vi "Create Rotated Ellipse.vi"(9 "aspect ratio":cluster{"x":dbl, "y":dbl}={"x"=1.0, "y"=0.8}, 11 "diameter points":T1) -> (3 "XY Graph":cluster{"X":dbl, "Y":dbl}[](graph))   [LabVIEW 2019]
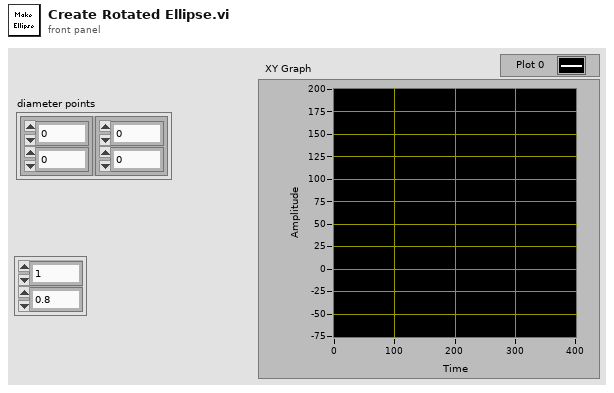
[diagram p1: front panel]
types:
  T1 = cluster{"first point":cluster{"x":dbl, "y":dbl}, "projected point":cluster{"x":dbl, "y":dbl}}
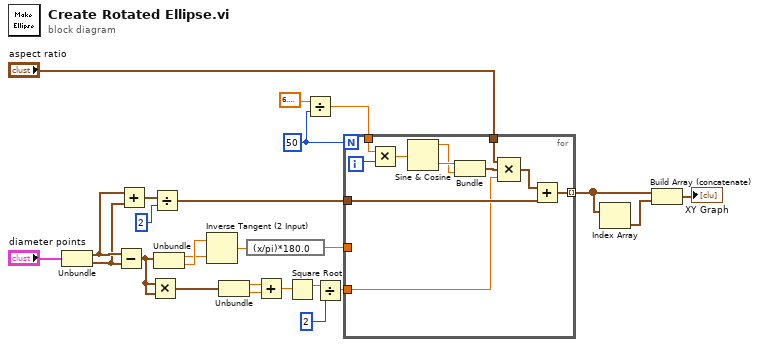
[diagram p0: block diagram]
diagram:
  w13 = 50
  n1 = Unbundle("diameter points") -> ("first point"=w22:cluster{"x":dbl, "y":dbl}, "projected point"=w21:cluster{"x":dbl, "y":dbl})
  n2 = Subtract(x=w22, y=w21) -> (x-y=w18:cluster{"x":dbl, "y":dbl})
  n3 = Add(x=w22, y=w21) -> (x+y=w20:cluster{"x":dbl, "y":dbl})
  n4 = Multiply(x=w18, y=w18) -> (x*y=w17:cluster{"x":dbl, "y":dbl})
  n5 = Divide(x=w20, y=2) -> (x/y=w15:cluster{"x":dbl, "y":dbl})
  n6 = Unbundle(w18) -> ("x"=w23:dbl, "y"=w24:dbl)
  n7 = Inverse Tangent (2 Input)(1:w23, 2:w24) -> (0:w3:dbl)
  n8 = Unbundle(w17) -> ("x"=w8:dbl, "y"=w7:dbl)
  n9 = expression code="(x/pi)*180.0" ("radians to degrees")(w3) -> (w2:dbl)
  n10 = Add(x=w8, y=w7) -> (x+y=w16:dbl)
  n11 = Square Root(x=w16) -> (sqrt(x)=w5:dbl)
  n12 = Divide(x=6.283185307179586, y=w13) -> (x/y=w12:dbl)
  n13 = Divide(x=w5, y=2) -> (x/y=w6:dbl)
  n14 = for {
    N: w13 -> [_]
    tunnel: w15 -> [w31]
    tunnel: w12 -> [w35]
    tunnel: [w30] -> w11 mode=indexing
    tunnel: w6 -> [w28]
    tunnel: w2 -> [_]
    tunnel: "aspect ratio" -> [w26]
    i -> [w36]
    n15 = Multiply(x=w35, y=w36) -> (x*y=w34:dbl)
    n16 = Sine & Cosine(0:w34) -> (1:w32:dbl, 2:w33:dbl)
    n17 = Bundle(w33, w32) -> (w29:cluster{dbl, dbl})  [unwired: 1 in]
    n18 = Compound Arithmetic op=MULTIPLY(w26, w29, w28) -> (w27:cluster{dbl, dbl})
    n19 = Add(x=w27, y=w31) -> (x+y=w30:cluster{dbl, dbl})
  }
  n20 = Index Array(array=w11) -> (element=w10:cluster{dbl, dbl})  [unwired: 1 in]
  n21 = Build Array (concatenate)(w11, w10) -> (→"XY Graph":cluster{dbl, dbl}[])
